vi "Saved Checker.vi"(1 "comp B":T7 {"?"."Limits"."StoopidFast (fps)" min=0.0; "?"."Limits"."Jerk (fps^3)" min=0.0 step=1.0; "?"."Limits"."Accel (fps^2)" min=0.0; "?"."Limits"."Velocity (fps)" min=0.0; "?"."Overrides"."Angle Override" step=5.0; "?"."Overrides"."Velocity Override" step=5.0; "?"."Overrides"."Angular Override" step=5.0; "?"."Angular Limits"."Jerk (deg/s^3)" min=0.0 step=1.0; "?"."Angular Limits"."Accel (deg/s^2)" min=0.0; "?"."Angular Limits"."Velocity (deg/s)" min=0.0}, 2 "comp A":T7 {"?"."Limits"."StoopidFast (fps)" min=0.0; "?"."Limits"."Jerk (fps^3)" min=0.0 step=1.0; "?"."Limits"."Accel (fps^2)" min=0.0; "?"."Limits"."Velocity (fps)" min=0.0; "?"."Overrides"."Angle Override" step=5.0; "?"."Overrides"."Velocity Override" step=5.0; "?"."Overrides"."Angular Override" step=5.0; "?"."Angular Limits"."Jerk (deg/s^3)" min=0.0 step=1.0; "?"."Angular Limits"."Accel (deg/s^2)" min=0.0; "?"."Angular Limits"."Velocity (deg/s)" min=0.0}, 3 "Save button ref":refnum<vi>) -> ()   [LabVIEW 2025]
uses:
  Types/Segment Type.ctl
  Types/Limits.ctl
  Types/Overrides.ctl
  Types/Angluar Limits.ctl
  Types/Single Cmd Info.ctl
  <vilib>/picture/picture.llb/imagedata.ctl
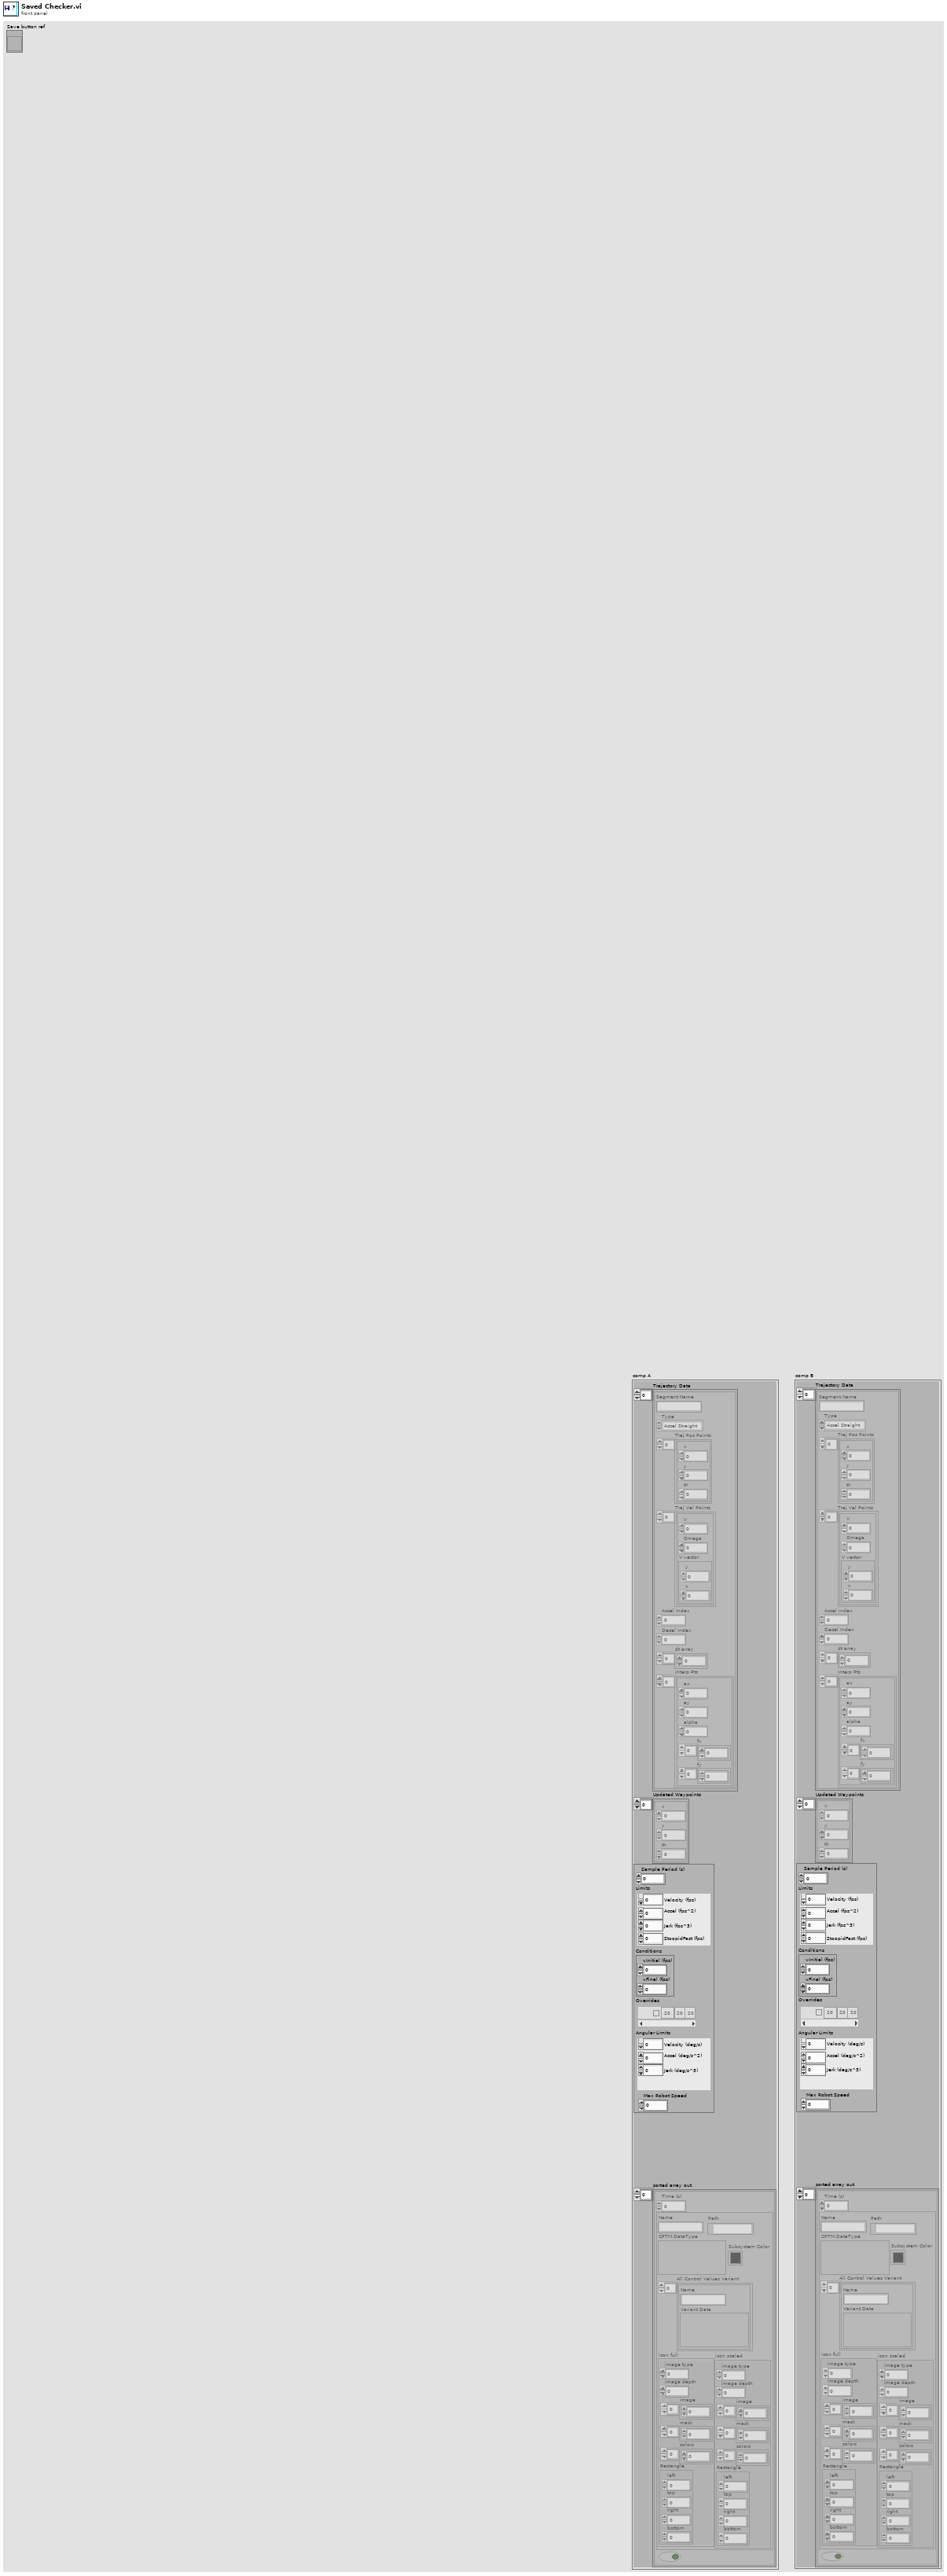
[diagram p1: front panel]
types:
  T1 = typedef "Segment Type.ctl" = enum16{"Accel Straight", "Const Straight", "Blend", "Circle", "Bezier", "Choreo"}
  T2 = typedef "Limits.ctl" = cluster{"Velocity (fps)":dbl, "Accel (fps^2)":dbl, "Jerk (fps^3)":dbl, "StoopidFast (fps)":dbl}
  T3 = typedef "Overrides.ctl" = cluster{"Count":string, "Angular Override":dbl, "Enabled?":bool, "Velocity Override":dbl, "Angle Override":dbl}[]
  T4 = typedef "Angluar Limits.ctl" = cluster{"Velocity (deg/s)":dbl, "Accel (deg/s^2)":dbl, "Jerk (deg/s^3)":dbl}
  T5 = typedef "Single Cmd Info.ctl" = cluster{"Name":string, "CPTM.DataType":variant, "All Control Values Variant":cluster{"Name":string, "Variant Data":variant}[], "icon full":T6, "icon scaled":T6, "Path":path, "Subsystem Color":u32}
  T6 = typedef "imagedata.ctl" = cluster{"image type":i32, "image depth":i32, "image":u8[], "mask":u8[], "colors":u32[], "Rectangle":cluster{"left":i16, "top":i16, "right":i16, "bottom":i16}}
  T7 = cluster{"Trajectory Data":cluster{"Segment Name":string, "Type":T1, "Traj Pos Points":cluster{"x":dbl, "y":dbl, "th":dbl}[], "Traj Vel Points":cluster{"V":dbl, "Omega":dbl, "V vector":cluster{"y":dbl, "x":dbl}}[], "Accel Index":i32, "Decel Index":i32, "dt array":dbl[], "Interp Pts":cluster{"ax":dbl, "ay":dbl, "alpha":dbl, "fx":dbl[], "fy":dbl[]}[]}[], "Updated Waypoints":cluster{"x":dbl, "y":dbl, "th":dbl}[], cluster{"Sample Period (s)":dbl, "Limits":T2, "Conditions":cluster{"vInitial (fps)":dbl, "vFinal (fps)":dbl}, "Overrides":T3, "Angular Limits":T4, "Max Robot Speed":dbl}, "sorted array out":cluster{"Time (s)":dbl, T5, bool}[]}
  T8 = cluster{"Segment Name":string, "Type":T1, "Traj Pos Points":cluster{"x":dbl, "y":dbl, "th":dbl}[], "Traj Vel Points":cluster{"V":dbl, "Omega":dbl, "V vector":cluster{"y":dbl, "x":dbl}}[], "Accel Index":i32, "Decel Index":i32, "dt array":dbl[], "Interp Pts":cluster{"ax":dbl, "ay":dbl, "alpha":dbl, "fx":dbl[], "fy":dbl[]}[]}[]
  T9 = cluster{"Sample Period (s)":dbl, "Limits":T2, "Conditions":cluster{"vInitial (fps)":dbl, "vFinal (fps)":dbl}, "Overrides":T3, "Angular Limits":T4, "Max Robot Speed":dbl}
  T10 = cluster{"V":dbl, "Omega":dbl, "V vector":cluster{"y":dbl, "x":dbl}}[]
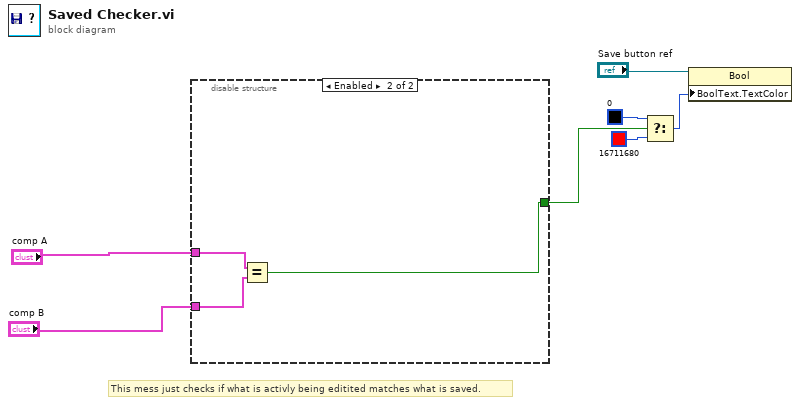
[diagram p0: block diagram]
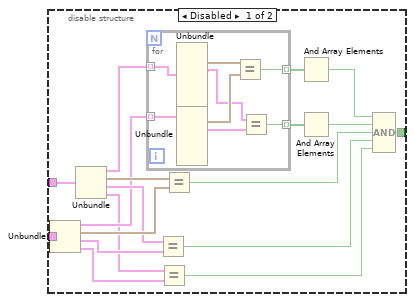
[diagram p2: hidden frame]
diagram:
  # "This mess just checks if what is activly being editited matches what is saved."
  n1 = disable-structure shown="Enabled" {
    disable-tunnel: [w10 w34] -> w3
    disable-tunnel: "comp B" -> [w9 w36]
    disable-tunnel: "comp A" -> [w8 w35]
    frame Disabled {
      n2 = Unbundle(w9) -> ("Trajectory Data"=w20:T8, "Updated Waypoints"=w24:cluster{"x":dbl, "y":dbl, "th":dbl}[], w21:T9, "sorted array out"=w13:cluster{"Time (s)":dbl, T5, bool}[])
      n3 = Unbundle(w8) -> ("Trajectory Data"=w22:T8, "Updated Waypoints"=w25:cluster{"x":dbl, "y":dbl, "th":dbl}[], w23:T9, "sorted array out"=w12:cluster{"Time (s)":dbl, T5, bool}[])
      n4 = for {
        tunnel: w22 -> [w33] mode=indexing
        tunnel: w20 -> [w32] mode=indexing
        tunnel: [w27] -> w19 mode=indexing
        tunnel: [w26] -> w18 mode=indexing
        n5 = Unbundle(w33) -> ("Traj Pos Points"=w31:cluster{"x":dbl, "y":dbl, "th":dbl}[], "Traj Vel Points"=w28:T10)  [unwired: 6 out]
        n6 = Unbundle(w32) -> ("Traj Pos Points"=w30:cluster{"x":dbl, "y":dbl, "th":dbl}[], "Traj Vel Points"=w29:T10)  [unwired: 6 out]
        n7 = Equal?(x=w31, y=w30) -> (x = y?=w27:bool)
        n8 = Equal?(x=w28, y=w29) -> (x = y?=w26:bool)
      }
      n9 = Equal?(x=w23, y=w21) -> (x = y?=w14:bool)
      n10 = Equal?(x=w12, y=w13) -> (x = y?=w11:bool)
      n11 = Equal?(x=w25, y=w24) -> (x = y?=w15:bool)
      n12 = And Array Elements(Boolean array=w19) -> (logical AND=w17:bool)
      n13 = And Array Elements(Boolean array=w18) -> (logical AND=w16:bool)
      n14 = Compound Arithmetic op=AND(w17, w16, w15, w14, w11) -> (w10:bool)
    }
    frame Enabled {
      n15 = Equal?(x=w35, y=w36) -> (x = y?=w34:bool)
    }
  }
  n16 = Select(t=u32 0 ("Boolean Text.Text Colors:Text Color"), s=w3, f=u32 16711680 ("Boolean Text.Text Colors:Text Color")) -> (s? t:f=w4:u32)
  n17 = property class="Bool"(reference="Save button ref", "BoolText.TextColor"=w4) -> ()  [unwired: 1 in, 2 out]
